vi "Reset Session.vi"(8 "error in (no error)":errorcluster, 11 "Session in":refnum<class "Session.lvclass">) -> (0 "error out":errorcluster, 3 "Session out":refnum<class "Session.lvclass">)   [LabVIEW 2020, in "HTTP Server.lvlib" / "Session.lvclass"]
uses:
  Session.lvclass
  Session.lvclass/Session.ctl
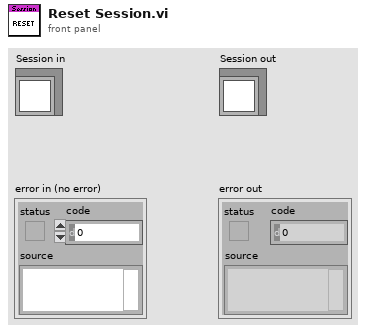
[diagram p1: front panel]
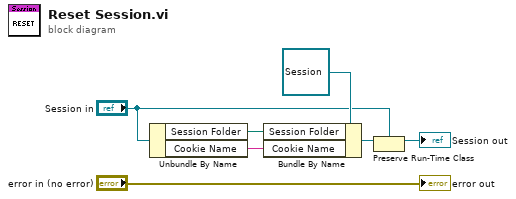
[diagram p0: block diagram]
diagram:
  n1 = Unbundle By Name("Session in") -> ("Session Folder"=w4:path, "Cookie Name"=w3:string)
  n2 = Bundle By Name(cluster=refnum<class "Session.lvclass"> refnum ("Session out"), "Session Folder"=w4, "Cookie Name"=w3) -> (w5:refnum<class "Session.lvclass">)
  n3 = Preserve Run-Time Class(object in=w5, 2:"Session in") -> (object out=→"Session out":refnum<class "Session.lvclass">)  [unwired: 1 in, 1 out]
  "error out" <- "error in (no error)"
